vi "ci-script.vi"() -> ()   [LabVIEW 2018]
uses:
  <resource>/Framework/Providers/InstaCoverage/Core/Defines/CoverageResult.ctl
  <resource>/Framework/Providers/InstaCoverage/Core/Defines/UserResultEnum.ctl
  <resource>/Framework/Providers/InstaCoverage/Core/Defines/TestReportTypeEnum.ctl
  <resource>/Framework/Providers/InstaCoverage/Core/TestSuite/Read CoverageResultEnum coverage.vi
  <resource>/Framework/Providers/InstaCoverage/Core/TestSuite/Read UserResultEnum.vi
  <resource>/Framework/Providers/InstaCoverage/Core/TestSuite/TestSuite.lvclass
  <resource>/Framework/Providers/InstaCoverage/Pro/InstaCoveragePro.lvlib
  <resource>/Framework/Providers/InstaCoverage/Core/InstaCoverageCore.lvlib
panel:
  out "files":T3(array[cluster])
  out "project":T3(array[cluster])
  out "Error Out":errorcluster
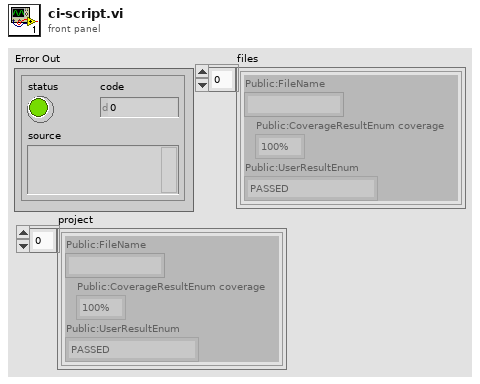
[diagram p1: front panel]
types:
  T1 = typedef "InstaCoverage.lvlib/InstaCoverageCore.lvlib/CoverageResult.ctl" = enum16{"100%", "NOT 100%", "N/A", "AVAILABLE IN PRO"}
  T2 = typedef "InstaCoverage.lvlib/InstaCoverageCore.lvlib/UserResultEnum.ctl" = enum16{"PASSED", "FAILED", "ERROR", "NONE", "AVAILABLE IN PRO"}
  T3 = cluster{"Public:FileName":string, "Public:CoverageResultEnum coverage":T1, "Public:UserResultEnum":T2}[]
  T4 = typedef "InstaCoverage.lvlib/InstaCoverageCore.lvlib/TestReportTypeEnum.ctl" = enum16{"JUNIT_XML", "HTML"}
  T5 = cluster{"Public:FileName":string, "Public:CoverageResultEnum coverage":T1, "Public:UserResultEnum":T2}
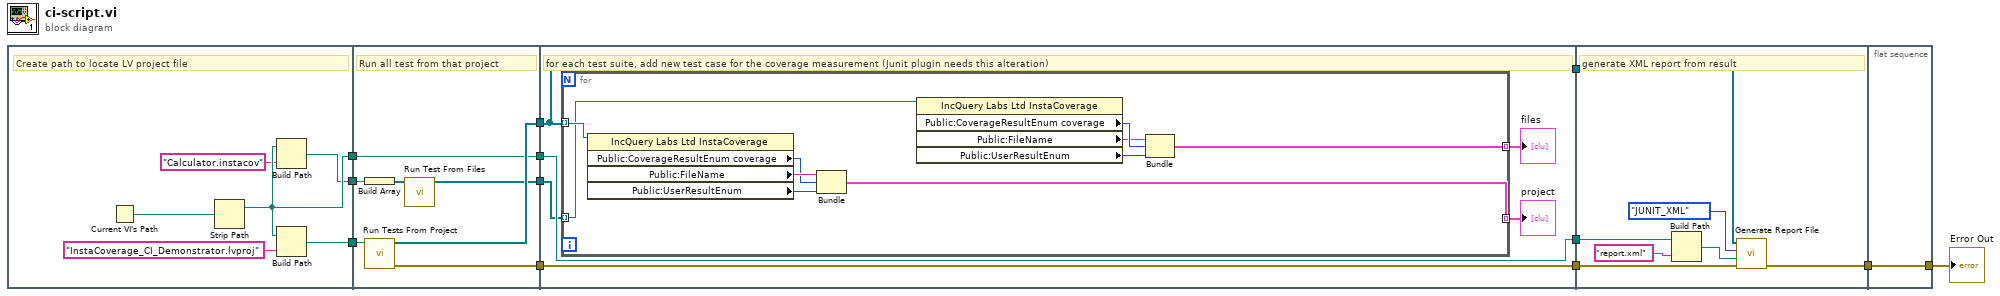
[diagram p0: block diagram]
diagram:
  n1 = flat-sequence {
    tunnel: [w16] -> w12
    tunnel: [w15] -> w9
    tunnel: [w13] -> w2
    tunnel: w12 -> [w25]
    tunnel: [w24] -> w11
    tunnel: [w23] -> w10
    tunnel: w9 -> [w22]
    tunnel: [w22] -> w8
    tunnel: w2 -> [w21]
    tunnel: [w19] -> w1
    tunnel: w11 -> [w30]
    tunnel: w10 -> [w29]
    tunnel: w8 -> [w31]
    tunnel: [w31] -> w7
    tunnel: [w30] -> w4
    tunnel: [w29] -> w3
    tunnel: w1 -> [w28]
    tunnel: w7 -> [w46]
    tunnel: [w43] -> w6
    tunnel: w4 -> [w48]
    tunnel: w3 -> [w42]
    tunnel: w6 -> [w49]
    tunnel: [w49] -> w5
    frame #0 {
      # "Create path to locate LV project file"
      n2 = Current VI's Path() -> (path=w18:path)
      n3 = Strip Path(path=w18) -> (stripped path=w15:path)  [unwired: 1 out]
      n4 = Build Path(base path=w15, name or relative path="Calculator.instacov") -> (appended path=w13:path)
      n5 = Build Path(base path=w15, name or relative path="InstaCoverage_CI_Demonstrator.lvproj") -> (appended path=w16:path)
    }
    frame #1 {
      # "Run all test from that project"
      n6 = Build Array(w21) -> (w20:path[])
      n7 = call <resource>:"Run Tests From Project.vi"("Path lvProject"=w25) -> ("Error out"=w24:errorcluster, "TestSuite[] results"=w23:refnum<class "TestSuite.lvclass">[])  [unwired: 9 in]
      n8 = call <resource>:"Run Test From Files.vi"("Path[] configs"=w20) -> ("TestSuite[] out"=w19:refnum<class "TestSuite.lvclass">[])  [unwired: 9 in, 1 out]
    }
    frame #2 {
      # "for each test suite, add new test case for the coverage measurement (Junit plugin needs this alteration)"
      n9 = for {
        tunnel: w29 -> [w41] mode=indexing
        tunnel: [w37] -> w27 mode=indexing
        tunnel: w28 -> [w33] mode=indexing
        tunnel: [w32] -> w26 mode=indexing
        n10 = property class="IncQuery Labs Ltd InstaCoverage"(reference=w41) -> ("Public:CoverageResultEnum coverage"=w39:T1, "Public:FileName"=w40:string, "Public:UserResultEnum"=w38:T2)  [unwired: 1 in, 2 out]
        n11 = Bundle("Public:FileName"=w40, "Public:CoverageResultEnum coverage"=w39, "Public:UserResultEnum"=w38) -> (w37:T5)  [unwired: 1 in]
        n12 = property class="IncQuery Labs Ltd InstaCoverage"(reference=w33) -> ("Public:CoverageResultEnum coverage"=w35:T1, "Public:FileName"=w34:string, "Public:UserResultEnum"=w36:T2)  [unwired: 1 in, 2 out]
        n13 = Bundle("Public:FileName"=w34, "Public:CoverageResultEnum coverage"=w35, "Public:UserResultEnum"=w36) -> (w32:T5)  [unwired: 1 in]
      }
      "project" <- w27
      "files" <- w26
    }
    frame #3 {
      # "generate XML report from result"
      n14 = Build Path(base path=w46, name or relative path="report.xml") -> (appended path=w44:path)
      n15 = call <resource>:"Generate Report File.vi"("Error In"=w48, "Path reportFile"=w44, "TestReportTypeEnum in"=TestReportTypeEnum."JUNIT_XML", "TestSuite[] in"=w42) -> ("Error Out"=w43:errorcluster)  [unwired: 7 in]
    }
    frame #4 {
    }
  }
  "Error Out" <- w5
